vi "microspec_validating.vi"() -> ()   [LabVIEW 2013]
uses:
  <vilib>/Instr/_visa.llb/VISA Configure Serial Port (Instr).vi
  <vilib>/Utility/file.llb/Write To Spreadsheet File (string).vi
panel:
  in  "Path":path
  in  "intergration time":dbl=54.0 caption="sensor\nintergration time (us)" min=54.0 max=5000000.0 step=100.0
  in  "?":T1(tab)=enum."measuring sequence"
  out "radiometer data file path":path
  in  "Runname":string
  out "Sensor_name":string="ILT1400"
  out "Radiometer Average":dbl
  in  "Delay":dbl=1.0
  in  "Step":dbl=1.0
  in  "Stop Wl":dbl=900.0 min=0.0 max=5000.0 step=100.0
  in  "Start Wl":dbl=300.0 min=0.0 max=5000.0 step=100.0
  in  "mean_number":i32=1 caption="Mean Number"
  out "Current Wavelength":dbl
  out "XY-Graph 2":cluster{"Y":dbl[], "Y":dbl[]}[](graph)
  in  "run 5":bool
  out "sectrometer data file path":path
  in  "save data":bool
  in  "reset with every wavelength?":bool caption="reset with new run?"
  in  "Delay":dbl=1.0
  in  "Step":dbl=10.0
  in  "Stop Wl":dbl=900.0 min=0.0 max=5000.0 step=100.0
  out "Current Wavelength":dbl
  in  "Start Wl 2":dbl=300.0 min=0.0 max=5000.0 step=10.0
  in  "Sensor":string(combo)="C12880MA_15B00040"
  in  "run 2":bool
  in  "Set Runs":i32=1
  out "Current Run":i32
  in  "stop runs":bool
  out "raw_data":cluster{"Y":dbl[], "Y":dbl[]}[](graph) caption="raw data"
  out "error":dbl
  out "raw_data 2":cluster{"Y":dbl[], "Y":dbl[]}[](graph) caption="raw data"
  in  "Stopp":bool
  out "System Setup":i32
  out "DLL Version":string
  out "Get Version":i32
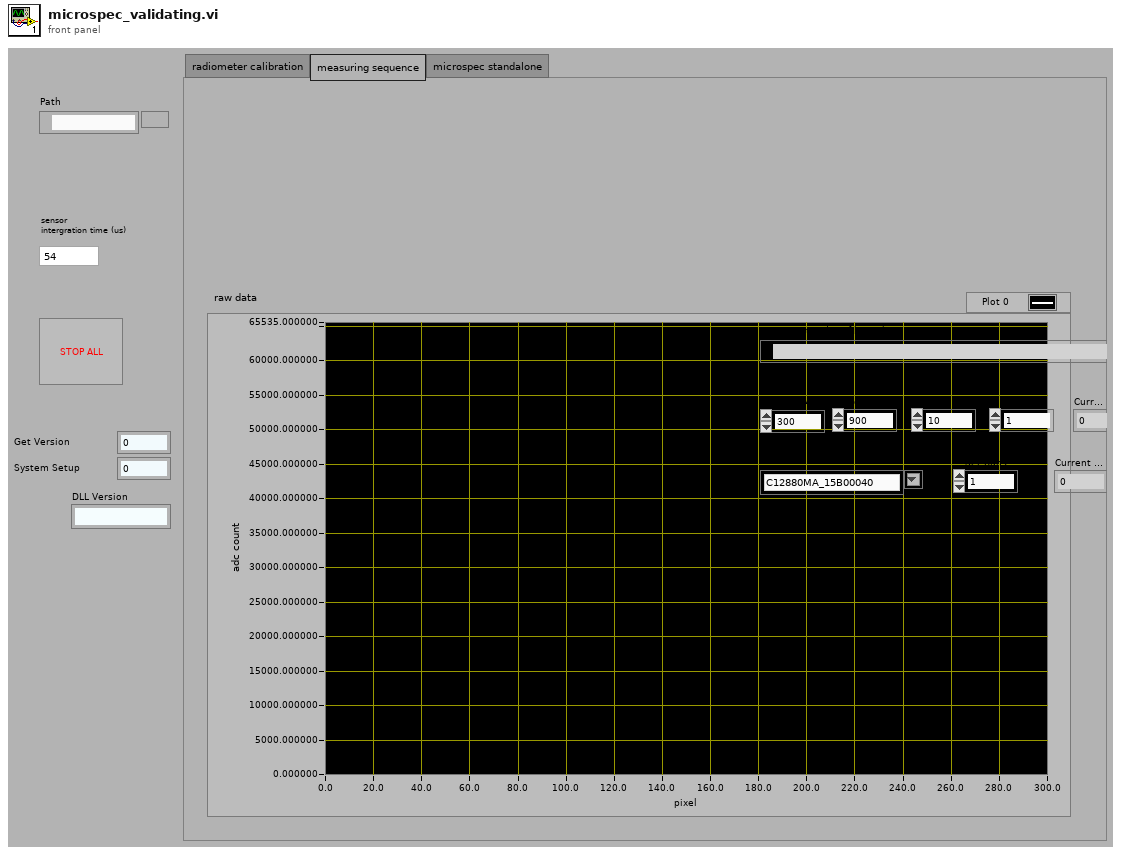
[diagram p1: front panel]
types:
  T1 = enum32{"radiometer calibration", "measuring sequence", "microspec standalone"}
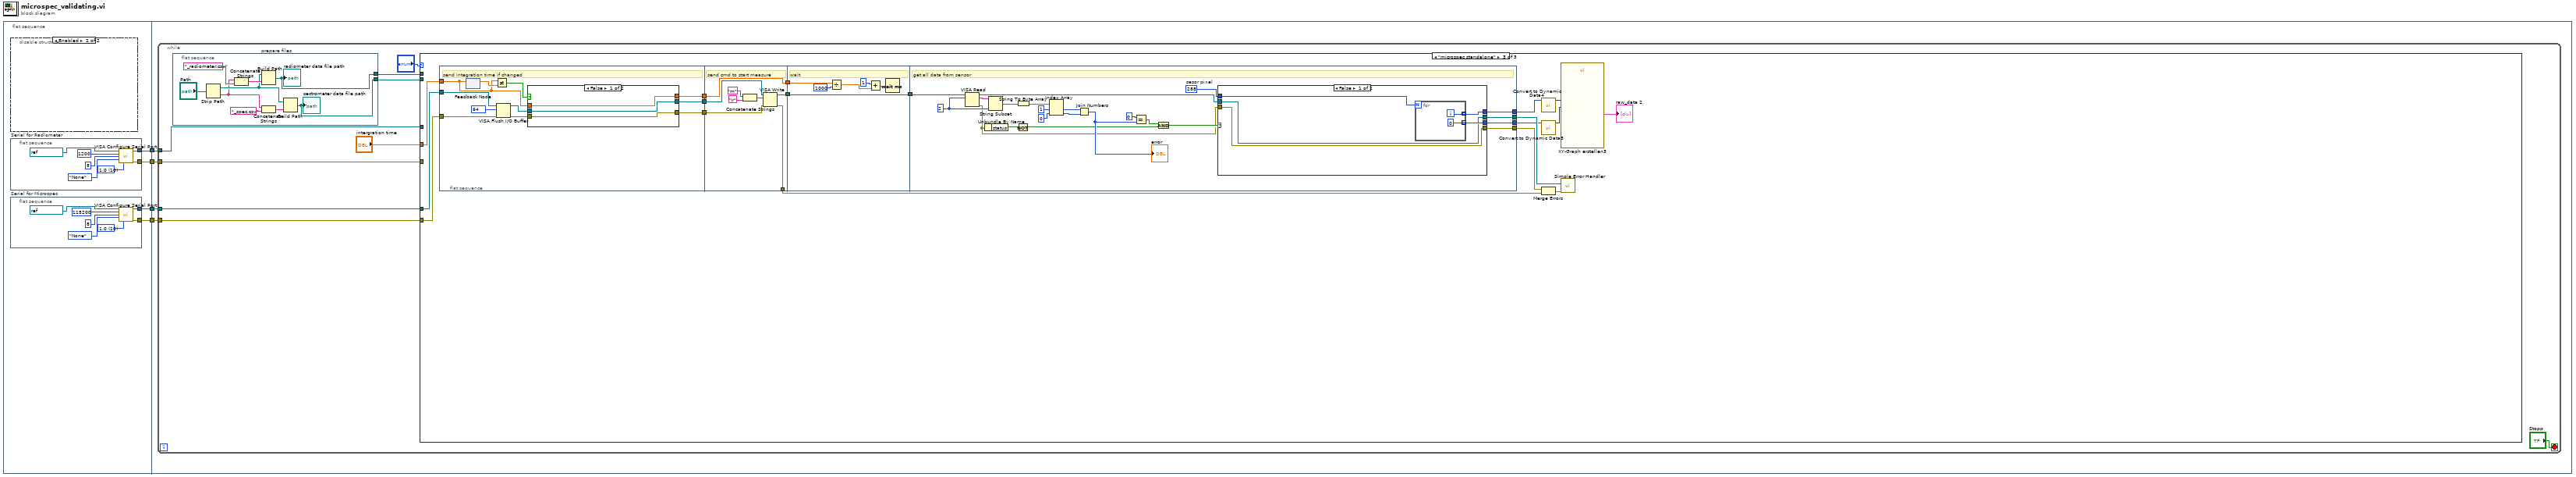
[diagram p0: block diagram]
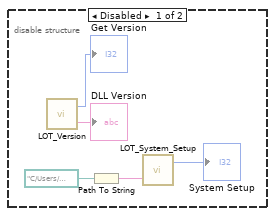
[diagram p2: hidden frame]
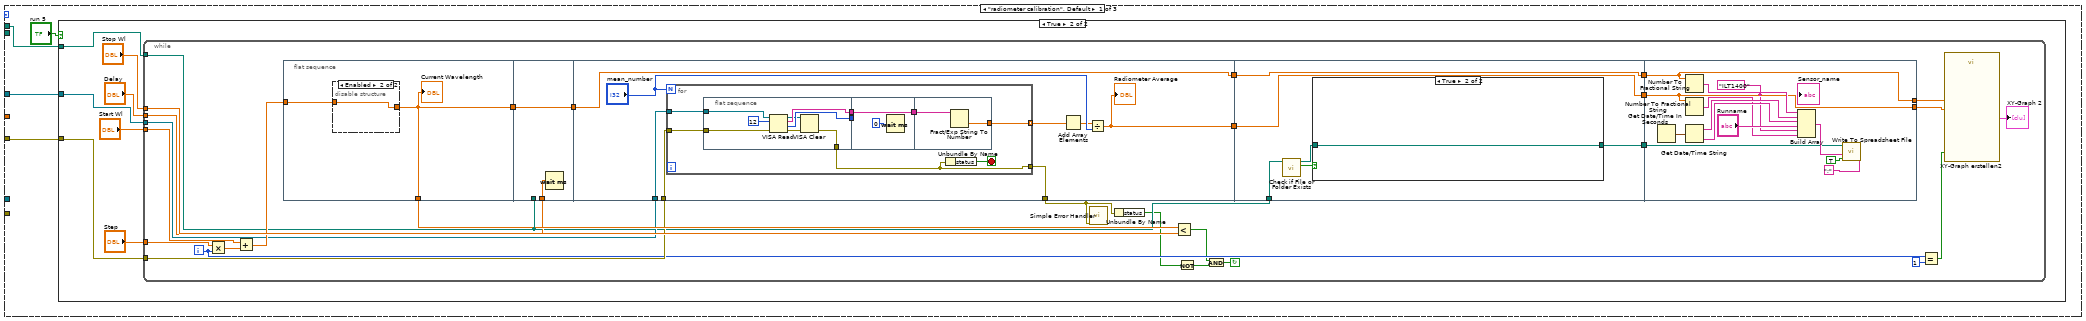
[diagram p3: hidden frame]
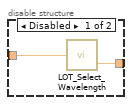
[diagram p5: hidden frame]
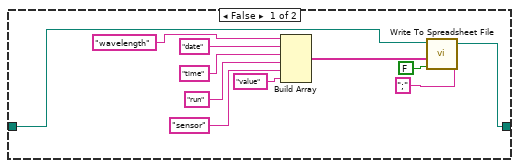
[diagram p6: hidden frame]
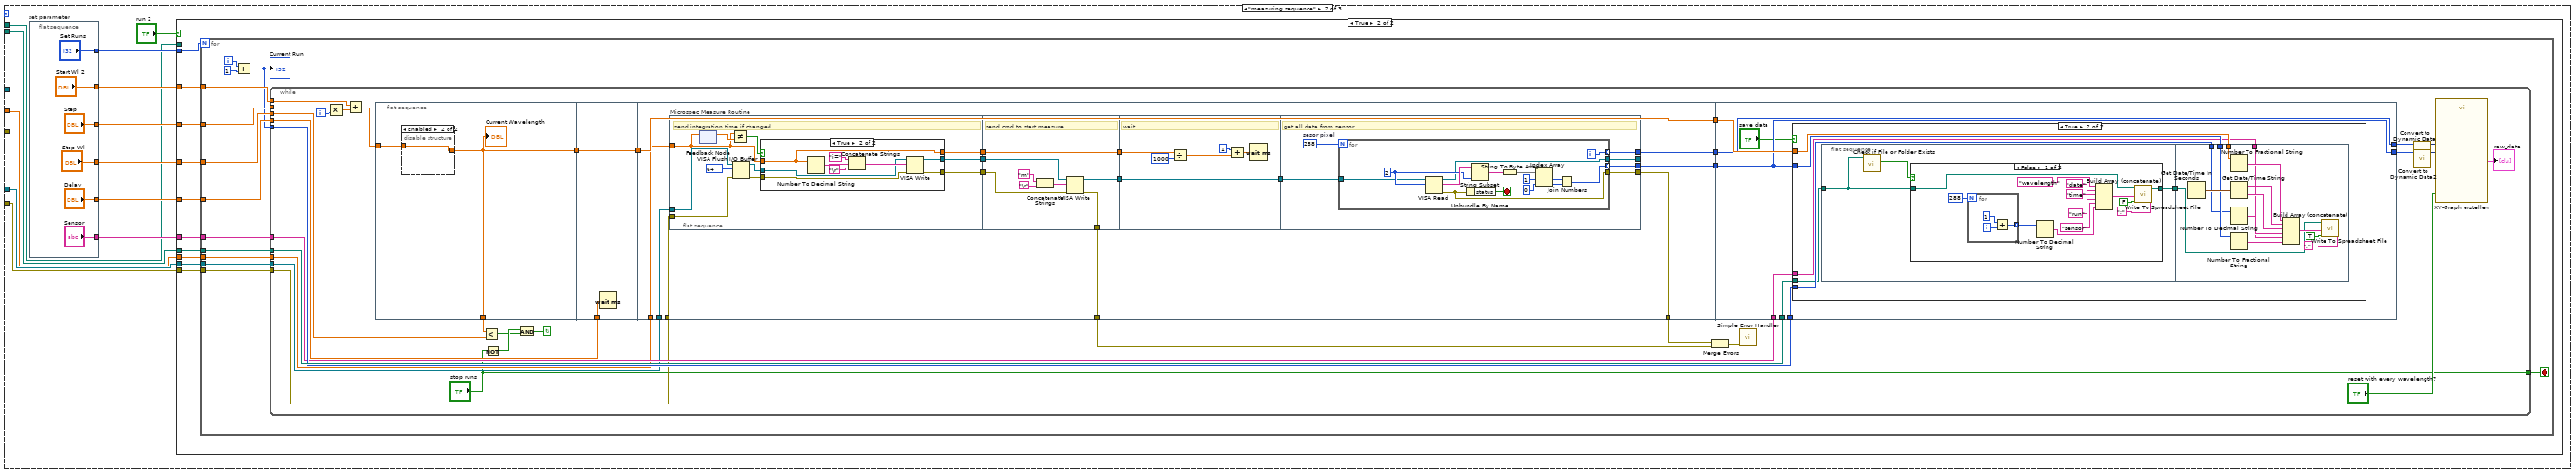
[diagram p7: hidden frame]
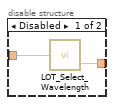
[diagram p9: hidden frame]
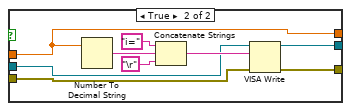
[diagram p13: hidden frame]
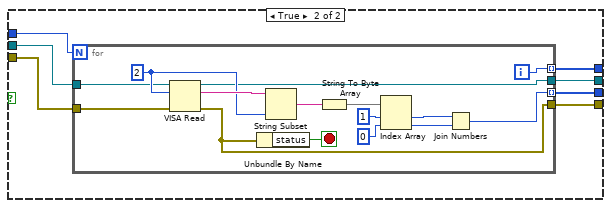
[diagram p14: hidden frame]
diagram:
  n1 = flat-sequence {
    tunnel: [w8] -> w4
    tunnel: [w7] -> w3
    tunnel: [w6] -> w2
    tunnel: [w5] -> w1
    tunnel: w4 -> [w31]
    tunnel: w3 -> [w30]
    tunnel: w2 -> [w29]
    tunnel: w1 -> [w28]
    frame #0 {
      # "Configuration"
      n2 = disable-structure shown="Enabled" {
        frame Disabled {
          n3 = call "LOT_Version.vi"() -> ("Version"=→"DLL Version":string, "Get Version"=→"Get Version":i32)
          n4 = Path To String(path=path "C:/Users/Public/Documents/LOT/Monochromator Control/Configurations/LOT_MSH-300_SN16578.xml" ("Configuration File")) -> (string=w25:string)
          n5 = call "LOT_System_Setup.vi"("CFG File Path"=w25) -> ("Error Code"=→"System Setup":i32)  [unwired: 2 in]
        }
        frame Enabled {
        }
      }
      n6 = flat-sequence "Serial for Radiometer" {
        tunnel: [w15] -> w6
        tunnel: [w14] -> w5
        frame #0 {
          w10 = u16 10 items=["1.0"=10, "1.5"=15, "2.0"=20] ("stop bits (10: 1 bit)")
          n7 = call-poly "VISA Configure Serial Port"("VISA resource name"=refnum<visa-resource-name> "COM4", "baud rate (9600)"=u32 1200, "data bits (8)"=u16 8, "parity (0:none)"=enum16{"None", "Odd", "Even", "Mark", "Space"}."None", "stop bits (10: 1 bit)"=w10) -> ("VISA resource name out"=w14:refnum<visa-resource-name>, "error out"=w15:errorcluster)  [unwired: 9 in]
        }
      }
      n8 = flat-sequence "Serial for Microspec" {
        tunnel: [w22] -> w8
        tunnel: [w21] -> w7
        frame #0 {
          w17 = u16 10 items=["1.0"=10, "1.5"=15, "2.0"=20] ("stop bits (10: 1 bit)")
          n9 = call-poly "VISA Configure Serial Port"("VISA resource name"=refnum<visa-resource-name> "COM11", "baud rate (9600)"=u32 115200, "data bits (8)"=u16 8, "parity (0:none)"=enum16{"None", "Odd", "Even", "Mark", "Space"}."None", "stop bits (10: 1 bit)"=w17) -> ("VISA resource name out"=w22:refnum<visa-resource-name>, "error out"=w21:errorcluster)  [unwired: 9 in]
        }
      }
    }
    frame #1 {
      n10 = while {
        tunnel: w31 -> [w38]
        tunnel: w30 -> [w37]
        tunnel: w29 -> [w36]
        tunnel: w28 -> [w35]
        stop <- "Stopp" stop-if-true
        n11 = flat-sequence "prepare files" {
          tunnel: [w41] -> w32
          tunnel: [w42] -> w33
          frame #0 {
            n12 = Strip Path(path="Path") -> (stripped path=w44:path, name=w43:string)
            n13 = Concatenate Strings(w43, "_radiometer.csv") -> (w45:string)
            n14 = Build Path(base path=w44, name or relative path=w45) -> (appended path=w42:path)
            "radiometer data file path" <- w42
            n15 = Concatenate Strings(w43, "_spec.csv") -> (w47:string)
            n16 = Build Path(base path=w44, name or relative path=w47) -> (appended path=w41:path)
            "sectrometer data file path" <- w41
          }
        }
        n17 = case shown="\"microspec standalone\"" "?" {
          tunnel: w32 -> [_ w165 _]
          tunnel: w38 -> [_ w164 w370]
          tunnel: w37 -> [_ w163 w369]
          tunnel: w36 -> [w52 _ _]
          tunnel: w35 -> [w51 _ _]
          tunnel: "intergration time" -> [_ w162 w368]
          tunnel: w33 -> [w50 w155 _]
          frame "radiometer calibration", Default {
            n18 = case shown="True" "run 5" {
              tunnel: w50 -> [_ w56]
              tunnel: w52 -> [_ w55]
              tunnel: w51 -> [_ w54]
              frame False {
              }
              frame True {
                n19 = while {
                  tunnel: "Step" -> [w88]
                  tunnel: "Start Wl" -> [w86]
                  tunnel: "Stop Wl" -> [w85]
                  tunnel: "Delay" -> [w81]
                  tunnel: w56 -> [w67]
                  tunnel: w54 -> [w80]
                  tunnel: w55 -> [w79]
                  i -> [w75]
                  stop <- w62 continue-if-true
                  n20 = Multiply(x=w88, y=w75) -> (x*y=w87:dbl)
                  n21 = Add(x=w86, y=w87) -> (x+y=w84:dbl)
                  n22 = flat-sequence {
                    tunnel: w84 -> [w90]
                    tunnel: [w89] -> w83
                    tunnel: [w89] -> w82
                    tunnel: w67 -> [_]
                    tunnel: w82 -> [w94]
                    tunnel: w81 -> [w95]
                    tunnel: [w94] -> w78
                    tunnel: w80 -> [w103]
                    tunnel: w79 -> [w102]
                    tunnel: w78 -> [w101]
                    tunnel: [w101] -> w71
                    tunnel: [w99] -> w69
                    tunnel: [w96] -> w61
                    tunnel: w71 -> [w129]
                    tunnel: [w129] -> w70
                    tunnel: w69 -> [w128]
                    tunnel: [w128] -> w68
                    tunnel: w67 -> [w126]
                    tunnel: [w127] -> w66
                    tunnel: [w145] -> w72
                    tunnel: [w146] -> w76
                    tunnel: w70 -> [w146]
                    tunnel: w68 -> [w145]
                    tunnel: w66 -> [w148]
                    frame #0 {
                      n23 = disable-structure shown="Enabled" {
                        disable-tunnel: w90 -> [w92 w93]
                        disable-tunnel: [w91 w93] -> w89
                        frame Disabled {
                          n24 = call "LOT_Select_Wavelength.vi"("Input Wavelength"=w92) -> ("Current Wavelength"=w91:dbl)  [unwired: 1 out]
                        }
                        frame Enabled {
                        }
                      }
                      "Current Wavelength" <- w89
                    }
                    frame #1 {
                      n25 = Wait (ms)(milliseconds to wait=w95) -> ()  [unwired: 1 out]
                    }
                    frame #2 {
                      n26 = for {
                        N: "mean_number" -> [_]
                        tunnel: w103 -> [w108]
                        tunnel: w102 -> [w107]
                        tunnel: [w106] -> w97 mode=indexing
                        tunnel: [w105] -> w96
                        stop <- w104 stop-if-true
                        n27 = flat-sequence {
                          tunnel: [w116] -> w111
                          tunnel: w108 -> [w119]
                          tunnel: w107 -> [w118]
                          tunnel: [w115] -> w110
                          tunnel: [w112] -> w105
                          tunnel: w111 -> [w121]
                          tunnel: [w121] -> w109
                          tunnel: w110 -> [_]
                          tunnel: w109 -> [w122]
                          tunnel: [w123] -> w106
                          frame #0 {
                            n28 = VISA Read(VISA resource name=w119, byte count=12, error in (no error)=w118) -> (VISA resource name out=w113:refnum<visa-resource-name>, read buffer=w116:string, return count=w115:u32, error out=w114:errorcluster)
                            n29 = VISA Clear(VISA resource name=w113, error in (no error)=w114) -> (error out=w112:errorcluster)  [unwired: 1 out]
                          }
                          frame #1 {
                            n30 = Wait (ms)(milliseconds to wait=u32 0 ("Zu wartende ms")) -> ()  [unwired: 1 out]
                          }
                          frame #2 {
                            n31 = Fract/Exp String To Number(string=w122) -> (number=w123:dbl)  [unwired: 3 in, 1 out]
                          }
                        }
                        n32 = Unbundle By Name(w105) -> ("status"=w104:bool)
                      }
                      n33 = Add Array Elements(numeric array=w97) -> (sum=w98:dbl)
                      n34 = Divide(x=w98, y="mean_number") -> (x/y=w99:dbl)
                      "Radiometer Average" <- w99
                    }
                    frame #3 {
                      n35 = call <vilib>:"Check if File or Folder Exists.vi"("path"=w126) -> ("file or folder exists?"=w125:bool, "dup path"=w124:path)  [unwired: 8 in, 1 out]
                      n36 = case shown="True" w125 {
                        tunnel: w124 -> [w138 w141]
                        tunnel: [w131 w141] -> w127
                        frame False {
                          n37 = Build Array("wavelength", "date" ("Element"), "time" ("Element"), "run" ("Element"), "sensor" ("Element"), "value") -> (w140:string[])
                          n38 = call-poly <vilib>:"Write To Spreadsheet File.vi"("delimiter (\\t)"=";", "append to file? (new file:F)"=FALSE, "1D data"=w140, "file path (dialog if empty)"=w138) -> ("new file path (Not A Path if cancelled)"=w131:path)  [unwired: 4 in]
                        }
                        frame True {
                        }
                      }
                    }
                    frame #4 {
                      w143 = "ILT1400" ("Sensor_name")
                      n39 = Get Date/Time In Seconds() -> (seconds since 1Jan1904=w153:timestamp)
                      n40 = Number To Fractional String(number=w146) -> (F-format string=w154:string)  [unwired: 3 in]
                      n41 = Number To Fractional String(number=w145) -> (F-format string=w142:string)  [unwired: 3 in]
                      n42 = Get Date/Time String(seconds (now)=w153) -> (date string=w152:string, time string=w151:string)  [unwired: 2 in]
                      n43 = Build Array(w154, w152, w151, "Runname", w143, w142) -> (w150:string[])
                      n44 = call-poly <vilib>:"Write To Spreadsheet File.vi"("delimiter (\\t)"=";", "append to file? (new file:F)"=TRUE, "1D data"=w150, "file path (dialog if empty)"=w148) -> ()  [unwired: 4 in, 1 out]
                      "Sensor_name" <- w143
                    }
                  }
                  n45 = call <vilib>:"Simple Error Handler.vi"("error in (no error)"=w61) -> ()  [unwired: 4 in, 5 out]
                  n46 = Unbundle By Name(w61) -> ("status"=w63:bool)
                  n47 = Less?(x=w83, y=w85) -> (x < y?=w65:bool)
                  n48 = Not(x=w63) -> (.not. x?=w64:bool)
                  n49 = And(x=w65, y=w64) -> (x .and. y?=w62:bool)
                  n50 = Equal?(x=w75, y=1) -> (x = y?=w73:bool)
                  n51 = call "XY-Graph erstellen2"("Reset"=w73, "Y Input"=w72, "X Input"=w76) -> ("XY Graph"=→"XY-Graph 2":cluster{"Y":dbl[], "Y":dbl[]}[])  [unwired: 7 in, 1 out]
                }
              }
            }
          }
          frame "measuring sequence" {
            n52 = flat-sequence "set parameter" {
              tunnel: ["Sensor"] -> w161
              tunnel: ["Delay"] -> w160
              tunnel: ["Step"] -> w159
              tunnel: ["Stop Wl"] -> w158
              tunnel: ["Start Wl 2"] -> w157
              tunnel: ["Set Runs"] -> w156
              frame #0 {
              }
            }
            n53 = case shown="True" "run 2" {
              tunnel: w165 -> [_ w173]
              tunnel: w161 -> [_ w182]
              tunnel: w156 -> [_ w181]
              tunnel: w164 -> [_ w180]
              tunnel: w163 -> [_ w179]
              tunnel: w160 -> [_ w178]
              tunnel: w158 -> [_ w177]
              tunnel: w159 -> [_ w176]
              tunnel: w157 -> [_ w175]
              tunnel: w162 -> [_ w174]
              tunnel: w155 -> [_ _]
              frame False {
              }
              frame True {
                n54 = for {
                  N: w181 -> [_]
                  tunnel: w173 -> [w195]
                  tunnel: w182 -> [w194]
                  tunnel: w180 -> [w193]
                  tunnel: w179 -> [w192]
                  tunnel: w178 -> [w191]
                  tunnel: w177 -> [w190]
                  tunnel: w176 -> [w189]
                  tunnel: w175 -> [w188]
                  tunnel: w174 -> [w187]
                  i -> [w186]
                  stop <- w183 stop-if-true
                  n55 = Add(x=w186, y=1) -> (x+y=w185:i32)
                  "Current Run" <- w185
                  n56 = while {
                    tunnel: w195 -> [w225]
                    tunnel: w185 -> [w224]
                    tunnel: w194 -> [w220]
                    tunnel: w193 -> [w218]
                    tunnel: w192 -> [w217]
                    tunnel: w191 -> [w208]
                    tunnel: w190 -> [w206]
                    tunnel: w189 -> [w205]
                    tunnel: w188 -> [w204]
                    tunnel: w187 -> [w203]
                    tunnel: ["stop runs"] -> w183
                    i -> [w222]
                    stop <- w197 continue-if-true
                    n57 = Multiply(x=w205, y=w222) -> (x*y=w227:dbl)
                    n58 = Add(x=w204, y=w227) -> (x+y=w226:dbl)
                    n59 = flat-sequence {
                      tunnel: w226 -> [w229]
                      tunnel: [w228] -> w223
                      tunnel: [w228] -> w207
                      tunnel: w223 -> [w233]
                      tunnel: w208 -> [w234]
                      tunnel: [w233] -> w211
                      tunnel: [w237] -> w219
                      tunnel: w218 -> [w241]
                      tunnel: w217 -> [w242]
                      tunnel: [w240] -> w215
                      tunnel: [w239] -> w214
                      tunnel: [w238] -> w213
                      tunnel: w211 -> [w237]
                      tunnel: w203 -> [w236]
                      tunnel: [w235] -> w202
                      tunnel: w225 -> [w312]
                      tunnel: w219 -> [w311]
                      tunnel: w224 -> [w310]
                      tunnel: [w308] -> w209
                      tunnel: w220 -> [w309]
                      tunnel: w213 -> [w308]
                      tunnel: w202 -> [w307]
                      tunnel: [w307] -> w201
                      frame #0 {
                        # "set wavelength"
                        n60 = disable-structure shown="Enabled" {
                          disable-tunnel: w229 -> [w231 w232]
                          disable-tunnel: [w230 w232] -> w228
                          frame Disabled {
                            n61 = call "LOT_Select_Wavelength.vi"("Input Wavelength"=w231) -> ("Current Wavelength"=w230:dbl)  [unwired: 1 out]
                          }
                          frame Enabled {
                          }
                        }
                        "Current Wavelength" <- w228
                      }
                      frame #1 {
                        # "wait"
                        n62 = Wait (ms)(milliseconds to wait=w234) -> ()  [unwired: 1 out]
                      }
                      frame #2 {
                        n63 = flat-sequence "Microspec Measure Routine" {
                          tunnel: w241 -> [w250]
                          tunnel: w242 -> [w259]
                          tunnel: [w254] -> w248
                          tunnel: [w253] -> w247
                          tunnel: [w252] -> w246
                          tunnel: w236 -> [w249]
                          tunnel: [w276] -> w245
                          tunnel: [w275] -> w239
                          tunnel: w248 -> [w273]
                          tunnel: w247 -> [w274]
                          tunnel: w246 -> [w272]
                          tunnel: [w272] -> w244
                          tunnel: w245 -> [w281]
                          tunnel: [w281] -> w243
                          tunnel: w244 -> [w280]
                          tunnel: w243 -> [w291]
                          tunnel: [w290] -> w238
                          tunnel: [w289] -> w235
                          tunnel: [w287] -> _
                          tunnel: [w286] -> w240
                          frame #0 {
                            # "send integration time if changed"
                            n64 = feedback #1() -> (w258:dbl)  [unwired: 1 in]
                            n65 = feedback-in #1(w249) -> ()
                            n66 = Not Equal?(x=w249, y=w258) -> (x != y?=w257:bool)
                            n67 = VISA Flush I/O Buffer(VISA resource name=w250, mask (16)=64, error in (no error)=w259) -> (VISA resource name out=w256:refnum<visa-resource-name>, error out=w255:errorcluster)
                            n68 = case shown="True" w257 {
                              tunnel: w256 -> [w261 w267]
                              tunnel: w255 -> [w260 w266]
                              tunnel: [w260 w265] -> w254
                              tunnel: [w261 w264] -> w253
                              tunnel: w249 -> [w262 w263]
                              tunnel: [w262 w263] -> w252
                              frame False {
                              }
                              frame True {
                                n69 = Number To Decimal String(number=w263) -> (decimal integer string=w270:string)  [unwired: 1 in]
                                n70 = Concatenate Strings("i=", w270, "\r") -> (w268:string)
                                n71 = VISA Write(VISA resource name=w267, write buffer=w268, error in (no error)=w266) -> (VISA resource name out=w264:refnum<visa-resource-name>, error out=w265:errorcluster)  [unwired: 1 out]
                              }
                            }
                          }
                          frame #1 {
                            # "send cmd to start measure"
                            n72 = Concatenate Strings("m", "\r") -> (w277:string)
                            n73 = VISA Write(VISA resource name=w274, write buffer=w277, error in (no error)=w273) -> (VISA resource name out=w276:refnum<visa-resource-name>, error out=w275:errorcluster)  [unwired: 1 out]
                          }
                          frame #2 {
                            # "wait"
                            n74 = Divide(x=w280, y=u32 1000 ("Zu wartende ms")) -> (x/y=w282:dbl)
                            n75 = Add(x=u32 1 ("Zu wartende ms"), y=w282) -> (x+y=w284:dbl)
                            n76 = Wait (ms)(milliseconds to wait=w284) -> ()  [unwired: 1 out]
                          }
                          frame #3 {
                            w288 = 288  # sesor pixel
                            # "get all data from sensor"
                            n77 = for {
                              N: w288 -> [_]
                              tunnel: w291 -> [w295]
                              tunnel: [w297] -> w290 mode=indexing
                              tunnel: [w296] -> w289 mode=indexing
                              tunnel: [w293] -> w287
                              tunnel: [w292] -> w286
                              i -> [w296]
                              stop <- w294 stop-if-true
                              w304 = 2
                              n78 = VISA Read(VISA resource name=w295, byte count=w304) -> (VISA resource name out=w293:refnum<visa-resource-name>, read buffer=w305:string, error out=w292:errorcluster)  [unwired: 1 in, 1 out]
                              n79 = Unbundle By Name(w292) -> ("status"=w294:bool)
                              n80 = String Subset(string=w305, length (rest)=w304) -> (substring=w303:string)  [unwired: 1 in]
                              n81 = String To Byte Array(string=w303) -> (unsigned byte array=w302:u8[])
                              n82 = Index Array(array=w302, index #1=1, index #2=0) -> (element #1=w298:u8, element #2=w299:u8)
                              n83 = Join Numbers(hi=w298, lo=w299) -> ((hi.lo)=w297:u16)
                            }
                          }
                        }
                      }
                      frame #3 {
                        n84 = case shown="True" "save data" {
                          tunnel: w312 -> [_ w315]
                          tunnel: w311 -> [_ w317]
                          tunnel: w310 -> [_ w316]
                          tunnel: w308 -> [_ w318]
                          tunnel: w309 -> [_ w314]
                          frame False {
                          }
                          frame True {
                            n85 = flat-sequence {
                              tunnel: w315 -> [w321]
                              tunnel: [w319] -> w313
                              tunnel: w318 -> [w345]
                              tunnel: w317 -> [w344]
                              tunnel: w316 -> [w343]
                              tunnel: w314 -> [w341]
                              tunnel: w313 -> [w339]
                              frame #0 {
                                n86 = call <vilib>:"Check if File or Folder Exists.vi"("path"=w321) -> ("file or folder exists?"=w320:bool)  [unwired: 8 in, 2 out]
                                n87 = case shown="False" w320 {
                                tunnel: w321 -> [w325 w338]
                                tunnel: [w322 w338] -> w319
                                frame False {
                                n88 = for {
                                N: 288 -> [_]
                                tunnel: [w335] -> w328 mode=indexing
                                i -> [w337]
                                n89 = Add(x=1, y=w337) -> (x+y=w335:i32)
                                }
                                n90 = Number To Decimal String(number=w328) -> (decimal integer string=w330:string[])  [unwired: 1 in]
                                n91 = Build Array (concatenate)("wavelength", "date" ("Element"), "time" ("Element"), "run" ("Element"), "sensor" ("Element"), w330) -> (w334:string[])
                                n92 = call-poly <vilib>:"Write To Spreadsheet File.vi"("delimiter (\\t)"=";", "append to file? (new file:F)"=FALSE, "1D data"=w334, "file path (dialog if empty)"=w325) -> ("new file path (Not A Path if cancelled)"=w322:path)  [unwired: 4 in]
                                }
                                frame True {
                                }
                                }
                              }
                              frame #1 {
                                n93 = Get Date/Time In Seconds() -> (seconds since 1Jan1904=w347:timestamp)
                                n94 = Number To Fractional String(number=w344) -> (F-format string=w346:string)  [unwired: 3 in]
                                n95 = Get Date/Time String(seconds (now)=w347) -> (date string=w348:string, time string=w349:string)  [unwired: 2 in]
                                n96 = Number To Decimal String(number=w343) -> (decimal integer string=w342:string)  [unwired: 1 in]
                                n97 = Number To Fractional String(number=w345) -> (F-format string=w352:string[])  [unwired: 3 in]
                                n98 = Build Array (concatenate)(w346, w348, w349, w342, w341, w352) -> (w350:string[])
                                n99 = call-poly <vilib>:"Write To Spreadsheet File.vi"("delimiter (\\t)"=";", "append to file? (new file:F)"=TRUE, "1D data"=w350, "file path (dialog if empty)"=w339) -> ()  [unwired: 4 in, 1 out]
                              }
                            }
                          }
                        }
                      }
                    }
                    n100 = Less?(x=w207, y=w206) -> (x < y?=w198:bool)
                    n101 = Not(x="stop runs") -> (.not. x?=w199:bool)
                    n102 = And(x=w199, y=w198) -> (x .and. y?=w197:bool)
                    n103 = Merge Errors(w215, w214) -> (w216:errorcluster)
                    n104 = call <vilib>:"Simple Error Handler.vi"("error in (no error)"=w216) -> ()  [unwired: 4 in, 5 out]
                    n105 = call "Convert to Dynamic Data"("Array"=w201) -> ("Dynamic Data Type"=w210:dynamicdata)  [unwired: 3 in]
                    n106 = call "Convert to Dynamic Data2"("Array"=w209) -> ("Dynamic Data Type"=w212:dynamicdata)  [unwired: 3 in]
                    n107 = call "XY-Graph erstellen"("Reset"="reset with every wavelength?", "Y Input"=w212, "X Input"=w210) -> ("XY Graph"=→"raw_data":cluster{"Y":dbl[], "Y":dbl[]}[])  [unwired: 7 in, 1 out]
                  }
                }
              }
            }
          }
          frame "microspec standalone" {
            n108 = flat-sequence {
              tunnel: w370 -> [w380]
              tunnel: w369 -> [w381]
              tunnel: [w375] -> w367
              tunnel: [w374] -> w366
              tunnel: [w373] -> w365
              tunnel: w368 -> [w371]
              tunnel: [w398] -> w364
              tunnel: [w397] -> w360
              tunnel: w367 -> [w395]
              tunnel: w366 -> [w396]
              tunnel: w365 -> [w394]
              tunnel: [w394] -> w363
              tunnel: w364 -> [w403]
              tunnel: [w403] -> w362
              tunnel: w363 -> [w402]
              tunnel: w362 -> [w416]
              tunnel: [w429] -> w361
              tunnel: [w428] -> w354
              tunnel: [w427] -> w353
              tunnel: [w425] -> w358
              frame #0 {
                # "send integration time if changed"
                n109 = feedback #2() -> (w379:dbl)  [unwired: 1 in]
                n110 = feedback-in #2(w371) -> ()
                n111 = Not Equal?(x=w371, y=w379) -> (x != y?=w378:bool)
                n112 = VISA Flush I/O Buffer(VISA resource name=w380, mask (16)=64, error in (no error)=w381) -> (VISA resource name out=w377:refnum<visa-resource-name>, error out=w376:errorcluster)
                n113 = case shown="False" w378 {
                  tunnel: w377 -> [w383 w389]
                  tunnel: w376 -> [w382 w388]
                  tunnel: [w382 w387] -> w375
                  tunnel: [w383 w386] -> w374
                  tunnel: w371 -> [w384 w385]
                  tunnel: [w384 w385] -> w373
                  frame False {
                  }
                  frame True {
                    n114 = Number To Decimal String(number=w385) -> (decimal integer string=w392:string)  [unwired: 1 in]
                    n115 = Concatenate Strings("i=", w392, "\r") -> (w390:string)
                    n116 = VISA Write(VISA resource name=w389, write buffer=w390, error in (no error)=w388) -> (VISA resource name out=w386:refnum<visa-resource-name>, error out=w387:errorcluster)  [unwired: 1 out]
                  }
                }
              }
              frame #1 {
                # "send cmd to start measure"
                n117 = Concatenate Strings("m", "\r") -> (w399:string)
                n118 = VISA Write(VISA resource name=w396, write buffer=w399, error in (no error)=w395) -> (VISA resource name out=w398:refnum<visa-resource-name>, error out=w397:errorcluster)  [unwired: 1 out]
              }
              frame #2 {
                # "wait"
                n119 = Divide(x=w402, y=u32 1000 ("Zu wartende ms")) -> (x/y=w404:dbl)
                n120 = Add(x=u32 1 ("Zu wartende ms"), y=w404) -> (x+y=w406:dbl)
                n121 = Wait (ms)(milliseconds to wait=w406) -> ()  [unwired: 1 out]
              }
              frame #3 {
                w423 = 2
                w426 = 288  # sesor pixel
                # "get all data from sensor"
                n122 = VISA Read(VISA resource name=w416, byte count=w423) -> (VISA resource name out=w415:refnum<visa-resource-name>, read buffer=w424:string, error out=w408:errorcluster)  [unwired: 1 in, 1 out]
                n123 = Unbundle By Name(w408) -> ("status"=w412:bool)
                n124 = String Subset(string=w424, length (rest)=w423) -> (substring=w422:string)  [unwired: 1 in]
                n125 = Not(x=w412) -> (.not. x?=w410:bool)
                n126 = String To Byte Array(string=w422) -> (unsigned byte array=w421:u8[])
                n127 = Index Array(array=w421, index #1=1, index #2=0) -> (element #1=w417:u8, element #2=w418:u8)
                n128 = Join Numbers(hi=w417, lo=w418) -> ((hi.lo)=w413:u16)
                "error" <- w413
                n129 = Equal?(x=0, y=w413) -> (x = y?=w409:bool)
                n130 = And(x=w409, y=w410) -> (x .and. y?=w411:bool)
                n131 = case shown="False" w411 {
                  tunnel: [w432 w443] -> w429
                  tunnel: w415 -> [w431 w442]
                  tunnel: [w433 w441] -> w428
                  tunnel: [w434 w440] -> w427
                  tunnel: w426 -> [w430 w439]
                  tunnel: [w431 w438] -> w425
                  tunnel: w408 -> [w432 w437]
                  frame False {
                    n132 = for {
                      N: w430 -> [_]
                      tunnel: [0] -> w433 mode=indexing
                      tunnel: [w436] -> w434 mode=indexing
                      i -> [w436]
                    }
                  }
                  frame True {
                    n133 = for {
                      N: w439 -> [_]
                      tunnel: w442 -> [w448]
                      tunnel: [w447] -> w443
                      tunnel: [w450] -> w441 mode=indexing
                      tunnel: [w449] -> w440 mode=indexing
                      tunnel: [w445] -> w438
                      tunnel: w437 -> [w444]
                      i -> [w449]
                      stop <- w446 stop-if-true
                      w457 = 2
                      n134 = VISA Read(VISA resource name=w448, byte count=w457, error in (no error)=w444) -> (VISA resource name out=w445:refnum<visa-resource-name>, read buffer=w458:string, error out=w447:errorcluster)  [unwired: 1 out]
                      n135 = Unbundle By Name(w447) -> ("status"=w446:bool)
                      n136 = String Subset(string=w458, length (rest)=w457) -> (substring=w456:string)  [unwired: 1 in]
                      n137 = String To Byte Array(string=w456) -> (unsigned byte array=w455:u8[])
                      n138 = Index Array(array=w455, index #1=1, index #2=0) -> (element #1=w451:u8, element #2=w452:u8)
                      n139 = Join Numbers(hi=w451, lo=w452) -> ((hi.lo)=w450:u16)
                    }
                  }
                }
              }
            }
            n140 = call "Convert to Dynamic Data4"("Array"=w353) -> ("Dynamic Data Type"=w355:dynamicdata)  [unwired: 3 in]
            n141 = call "Convert to Dynamic Data3"("Array"=w354) -> ("Dynamic Data Type"=w356:dynamicdata)  [unwired: 3 in]
            n142 = Merge Errors(w361, w360) -> (w359:errorcluster)
            n143 = call "XY-Graph erstellen3"("Y Input"=w356, "X Input"=w355) -> ("XY Graph"=→"raw_data 2":cluster{"Y":dbl[], "Y":dbl[]}[])  [unwired: 8 in, 1 out]
            n144 = call <vilib>:"Simple Error Handler.vi"("error source (\" \")"=w358, "error in (no error)"=w359) -> ()  [unwired: 3 in, 5 out]
          }
        }
      }
    }
  }
